vi "Exemple_Metrics_Fowlkes_Mallows_Score.vi"() -> ()   [LabVIEW 2020]
uses:
  Objet/3 - Model selection and evaluation/3.3 - Metrics and scoring/fowlkes_mallows_score/Fowlkes_Mallows_Score.vi
panel:
  out "Score":string
  out "error out":errorcluster caption="sortie d'erreur"
  in  "fowlkes_mallows_score":cluster{"sparse":bool}
  in  "error in (no error)":errorcluster caption="entrée d'erreur (pas d'erreur)"
  in  "labels_pred":string[][](array[string])=[["0"], ["0"], ["1"], ["1"]]
  in  "labels_true":string[][](array[string])=[["0"], ["0"], ["1"], ["1"]]
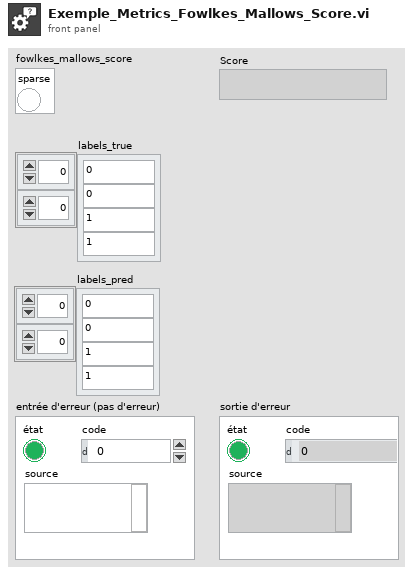
[diagram p1: front panel]
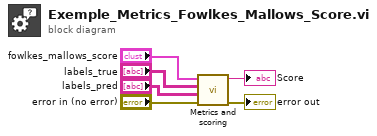
[diagram p0: block diagram]
diagram:
  n1 = call-poly "Metrics and scoring.vi"("error in (no error)"="error in (no error)", "labels_pred"="labels_pred", "labels_true"="labels_true", "fowlkes_mallows_score"="fowlkes_mallows_score") -> ("error out"=→"error out":errorcluster, "String Data"=→"Score":string)  [unwired: 6 in]
